vi "Read Earnings (dollars).vi"(8 "error in (no error)":errorcluster, 11 "Sports Player in":refnum<class "Sports Player.lvclass">) -> (0 "error out":errorcluster, 2 "Earnings (dollars)":dbl, 3 "Sports Player out":refnum<class "Sports Player.lvclass">)   [LabVIEW 2019, in "Sports Player.lvclass"]
uses:
  Sports Player.lvclass
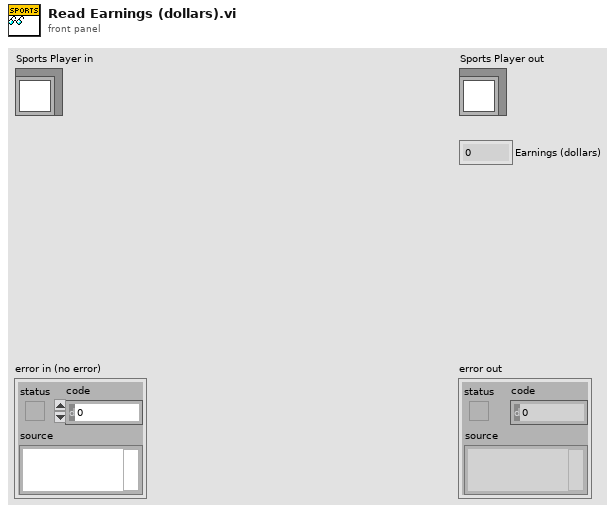
[diagram p1: front panel]
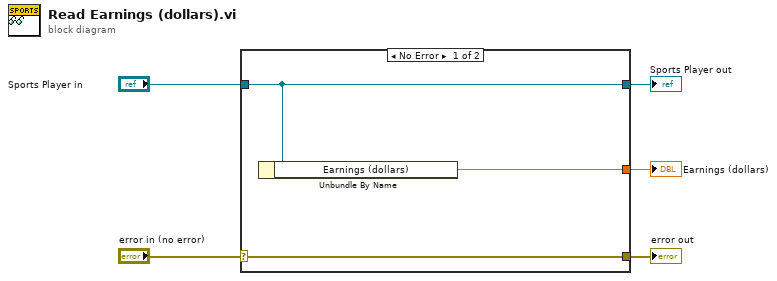
[diagram p0: block diagram]
diagram:
  n1 = case shown="No Error" "error in (no error)" {
    selector: "error in (no error)" -> [w8 w9]
    tunnel: [w8 w9] -> w4
    tunnel: [w7 w10] -> w2
    tunnel: "Sports Player in" -> [w7 w10]
    tunnel: [w6 _] -> w1
    frame No Error {
      n2 = Unbundle By Name(w7) -> ("Earnings (dollars)"=w6:dbl)
    }
    frame Error {
    }
  }
  "error out" <- w4
  "Sports Player out" <- w2
  "Earnings (dollars)" <- w1
